vi "onComputeIntervals.vi"(8 "error in (no error)":errorcluster, 9 "Cron Interval":T1, 10 "Expression":string, 11 "Cron.Quartz in":refnum<class "Cron.Quartz.lvclass">) -> (0 "error out":errorcluster, 2 "Interval Parameters":T2, 3 "Cron.Quartz out":refnum<class "Cron.Quartz.lvclass">)   [LabVIEW 2013, in "openCron.lvlib" / "Cron.Quartz.lvclass"]
uses:
  Cron.Quartz.lvclass
  Cron/Cron Interval -- cluster.ctl
  Cron/Cron Interval -- enum.ctl
  Cron/Cron.lvclass
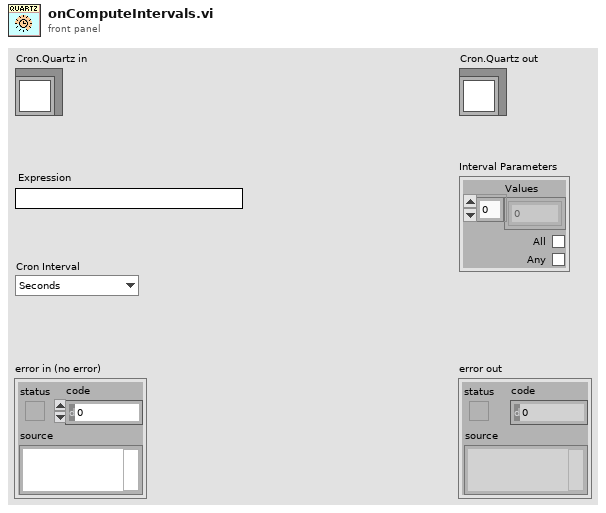
[diagram p1: front panel]
types:
  T1 = typedef "openCron.lvlib/Cron.lvclass/Cron Interval -- enum.ctl" = enum16{"Seconds", "Minutes", "Hours", "Day of Month", "Month", "Day of Week", "Year"}
  T2 = typedef "openCron.lvlib/Cron.lvclass/Cron Interval -- cluster.ctl" = cluster{"Values":i32[], "All":bool, "Any":bool}
  T3 = enum16{"SUN", "MON", "TUE", "WED", "THU", "FRI", "SAT"}
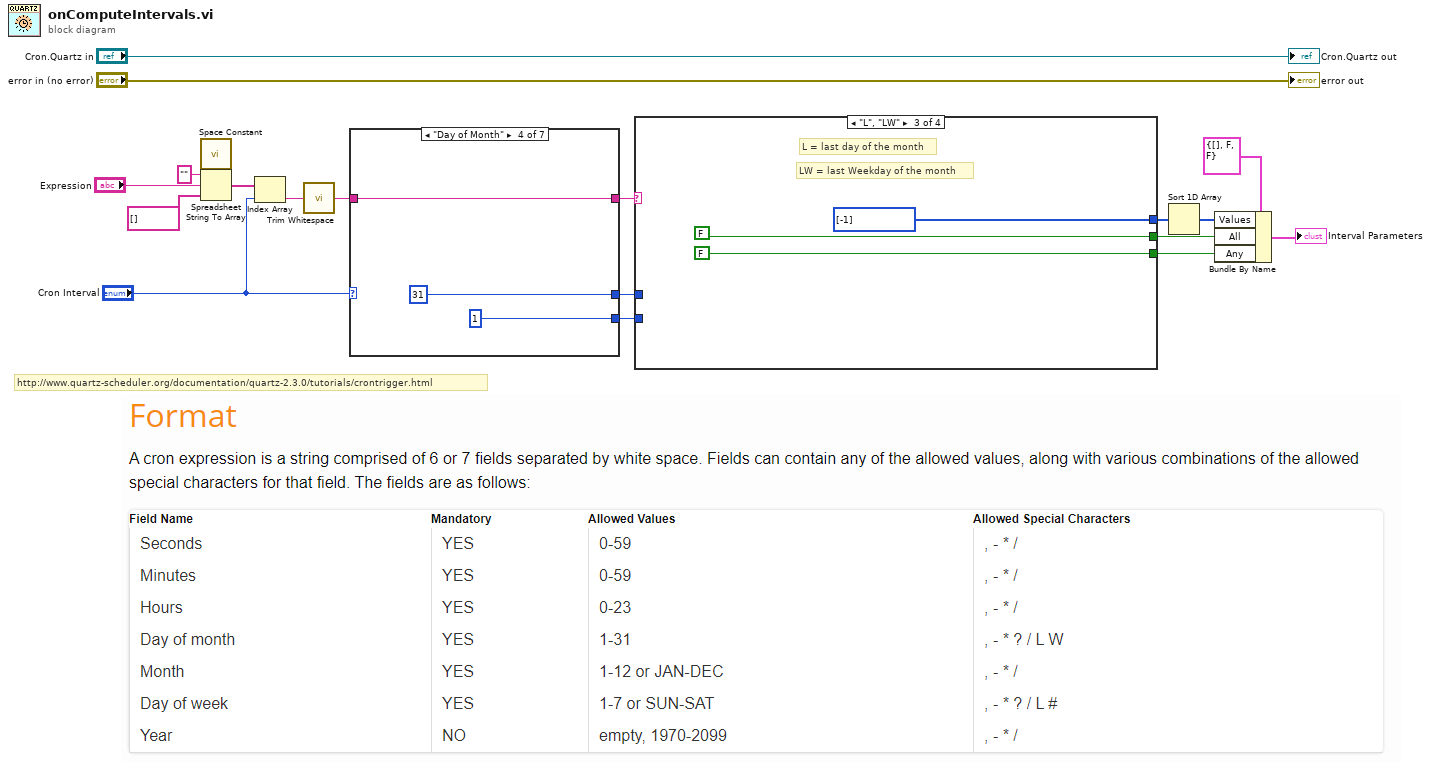
[diagram p0: block diagram]
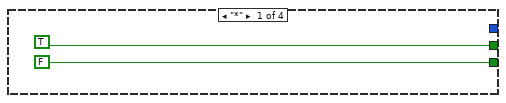
[diagram p2: hidden frame]
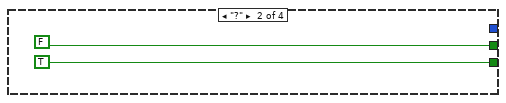
[diagram p3: hidden frame]
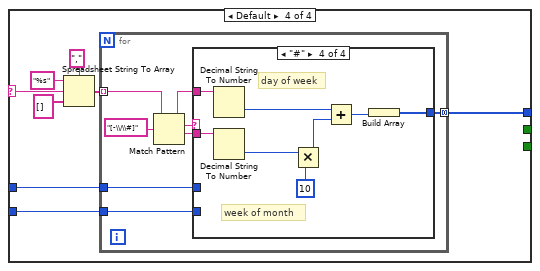
[diagram p4: hidden frame]
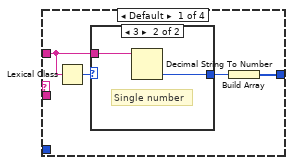
[diagram p5: hidden frame]
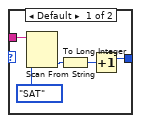
[diagram p6: hidden frame]
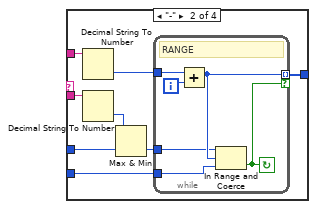
[diagram p7: hidden frame]
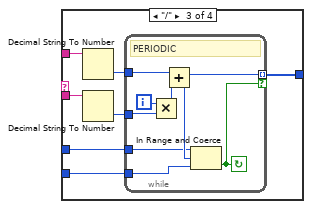
[diagram p8: hidden frame]
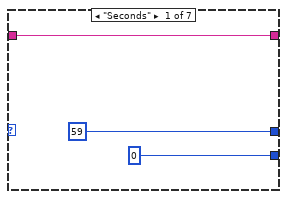
[diagram p9: hidden frame]
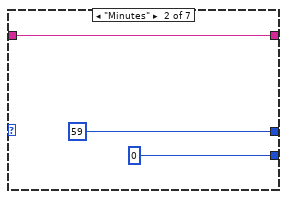
[diagram p10: hidden frame]
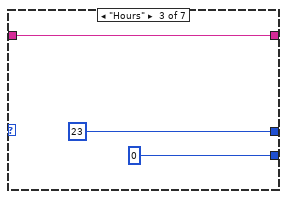
[diagram p11: hidden frame]
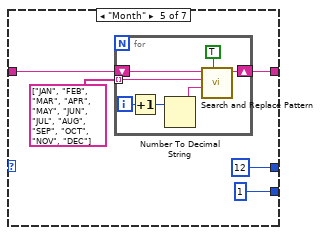
[diagram p12: hidden frame]
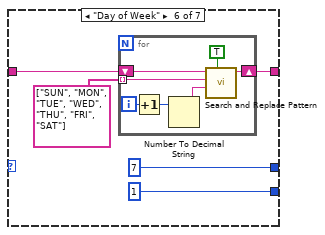
[diagram p13: hidden frame]
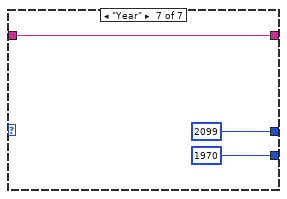
[diagram p14: hidden frame]
diagram:
  # "http://www.quartz-scheduler.org/documentation/quartz-2.3.0/tutorials/crontrigger.html"
  n1 = call <vilib>:"Space Constant.vi"() -> ("String"=w14:string)
  n2 = Spreadsheet String To Array(delimiter (Tab)=w14, format string="", spreadsheet string="Expression", array type (2D Dbl)=string[] []) -> (array=w13:string[])
  n3 = Index Array(array=w13, index="Cron Interval") -> (element=w11:string)
  n4 = call <vilib>:"Trim Whitespace.vi"("string"=w11) -> ("trimmed string"=w2:string)  [unwired: 1 in]
  n5 = case shown="\"Day of Month\"" "Cron Interval" {
    tunnel: [59 ("y") 59 ("y") 23 ("y") 31 ("y") 12 ("y") 7 ("y") 2099 ("y")] -> w10
    tunnel: [0 ("y") 0 ("y") 0 ("y") 1 ("y") 1 ("y") 1 ("y") 1970 ("y")] -> w9
    tunnel: w2 -> [w20 w23 w26 w29 w33 w45 w56]
    tunnel: [w20 w23 w26 w29 w34 w44 w56] -> w1
    frame "Seconds" {
    }
    frame "Minutes" {
    }
    frame "Hours" {
    }
    frame "Day of Month" {
    }
    frame "Month" {
      n6 = for {
        shift-right: [w43] -> w34
        shift-left: w33 -> [w42]
        tunnel: string[] ["JAN", "FEB", "MAR", "APR", "MAY", "JUN", "JUL", "AUG", "SEP", "OCT", "NOV", "DEC"] -> [w40] mode=indexing
        i -> [w39]
        n7 = Increment(x=w39) -> (x+1=w38:i32)
        n8 = Number To Decimal String(number=w38) -> (decimal integer string=w37:string)  [unwired: 1 in]
        n9 = call <vilib>:"Search and Replace Pattern.vi"("string"=w42, "regular expression (\"\")"=w40, "replace string (\"\")"=w37, "replace all? (F)"=TRUE) -> ("result string"=w43:string)  [unwired: 1 in, 1 out]
      }
    }
    frame "Day of Week" {
      n10 = for {
        shift-right: [w55] -> w44
        shift-left: w45 -> [w54]
        tunnel: string[] ["SUN", "MON", "TUE", "WED", "THU", "FRI", "SAT"] -> [w52] mode=indexing
        i -> [w51]
        n11 = Increment(x=w51) -> (x+1=w50:i32)
        n12 = Number To Decimal String(number=w50) -> (decimal integer string=w49:string)  [unwired: 1 in]
        n13 = call <vilib>:"Search and Replace Pattern.vi"("string"=w54, "regular expression (\"\")"=w52, "replace string (\"\")"=w49, "replace all? (F)"=TRUE) -> ("result string"=w55:string)  [unwired: 1 in, 1 out]
      }
    }
    frame "Year" {
    }
  }
  n14 = case shown="\"L\", \"LW\"" w1 {
    selector: w1 -> [_ _ _ w69]
    tunnel: [_ _ i32[] [-1] w68] -> w7
    tunnel: [TRUE FALSE FALSE _] -> w6
    tunnel: [FALSE TRUE FALSE _] -> w5
    tunnel: w10 -> [_ _ _ w67]
    tunnel: w9 -> [_ _ _ w66]
    frame "*" {
    }
    frame "?" {
    }
    frame "L", "LW" {
      # "L = last day of the month"
      # "LW = last Weekday of the month"
    }
    frame Default {
      n15 = Spreadsheet String To Array(delimiter (Tab)=",", format string="%s", spreadsheet string=w69, array type (2D Dbl)=string[] []) -> (array=w70:string[])
      n16 = for {
        tunnel: w70 -> [w81] mode=indexing
        tunnel: [w77] -> w68 mode=concatenating
        tunnel: w67 -> [w75]
        tunnel: w66 -> [w74]
        n17 = Match Pattern(string=w81, regular expression="[-\\/\\#]") -> (before substring=w78:string, match substring=w79:string, after substring=w76:string)  [unwired: 1 in, 1 out]
        n18 = case shown="\"#\"" w79 {
          tunnel: w78 -> [w83 w100 w113 w129]
          tunnel: [w84 w97 w111 w127] -> w77
          tunnel: w76 -> [_ w98 w109 w128]
          tunnel: w75 -> [_ w95 w108 _]
          tunnel: w74 -> [_ w94 w107 _]
          frame Default {
            n19 = Lexical Class(1:w83) -> (0:w82:i16)
            n20 = case shown="3" w82 {
              tunnel: [w86 w92] -> w85
              tunnel: w83 -> [w90 w91]
              frame Default {
                n21 = Scan From String(input string=w90, default 1=T3."SAT" ("y")) -> (output 1=w87:T3)  [unwired: 3 in, 3 out]
                n22 = To Long Integer(number=w87) -> (32bit integer=w88:i32)
                n23 = Increment(x=w88) -> (x+1=w86:i32)
              }
              frame 3 {
                # "Single number"
                n24 = Decimal String To Number(string=w91) -> (number=w92:i32)  [unwired: 2 in, 1 out]
              }
            }
            n25 = Build Array(w85) -> (w84:i32[])
          }
          frame "-" {
            n26 = Decimal String To Number(string=w100) -> (number=w99:i32)  [unwired: 2 in, 1 out]
            n27 = Decimal String To Number(string=w98) -> (number=w96:i32)  [unwired: 2 in, 1 out]
            n28 = Max & Min(x=w96, y=w95) -> (min(x,y)=w93:i32)  [unwired: 1 out]
            n29 = while {
              tunnel: w99 -> [w106]
              tunnel: [w103] -> w97 mode=indexing if=w104
              tunnel: w94 -> [w102]
              tunnel: w93 -> [w101]
              i -> [w105]
              stop <- w104 continue-if-true
              # "RANGE"
              n30 = Add(x=w106, y=w105) -> (x+y=w103:i32)
              n31 = In Range and Coerce(upper limit=w101, x=w103, lower limit=w102) -> (In Range?=w104:bool)  [unwired: 1 out]
            }
          }
          frame "/" {
            n32 = Decimal String To Number(string=w113) -> (number=w112:i32)  [unwired: 2 in, 1 out]
            n33 = Decimal String To Number(string=w109) -> (number=w110:i32)  [unwired: 2 in, 1 out]
            n34 = while {
              tunnel: w112 -> [w121]
              tunnel: [w117] -> w111 mode=indexing if=w114
              tunnel: w110 -> [w120]
              tunnel: w108 -> [w116]
              tunnel: w107 -> [w115]
              i -> [w119]
              stop <- w114 continue-if-true
              # "PERIODIC"
              n35 = Multiply(x=w119, y=w120) -> (x*y=w118:i32)
              n36 = Add(x=w121, y=w118) -> (x+y=w117:i32)
              n37 = In Range and Coerce(upper limit=w116, x=w117, lower limit=w115) -> (In Range?=w114:bool)  [unwired: 1 out]
            }
          }
          frame "#" {
            # "week of month"
            # "day of week"
            n38 = Decimal String To Number(string=w129) -> (number=w124:i32)  [unwired: 2 in, 1 out]
            n39 = Decimal String To Number(string=w128) -> (number=w126:i32)  [unwired: 2 in, 1 out]
            n40 = Multiply(x=w126, y=10) -> (x*y=w123:i32)
            n41 = Add(x=w124, y=w123) -> (x+y=w122:i32)
            n42 = Build Array(w122) -> (w127:i32[])
          }
        }
      }
    }
  }
  n43 = Sort 1D Array(array=w7) -> (sorted array=w8:i32[])
  n44 = Bundle By Name(cluster=T2 {"Values"=[], "All"=FALSE, "Any"=FALSE} ("Interval"), "Values"=w8, "All"=w6, "Any"=w5) -> (→"Interval Parameters":T2)
  "error out" <- "error in (no error)"
  "Cron.Quartz out" <- "Cron.Quartz in"
